vi "VPA QC Print Page.vi"(10 "State Cluster":T1) -> ()   [LabVIEW 2013]
uses:
  Controls/VPA QC General Cluster.ctl
  Controls/VPA QC State Data Cluster.ctl
  Controls/VPA QC State Enum.ctl
  Controls/VPA QC Bool Cluster.ctl
panel:
  out "Cyl B Const":dbl
  out "Cyl A Const.":dbl
  out "Wrap":bool caption="Wrap pump in plastic visqueen."
  out "Clean Water Out":bool caption="Take off the manifold and clear all water out of the\ncylinders and manifold"
  out "Maintenance Hours":bool caption="Reset Maintenance hours from the initial setup menu."
  out "Initialize Pump":bool caption="Initilaize pump to get the top position."
  out "Box":bool caption="Place VPA in box and all other required parts"
  out "Screws":bool caption="Verify that all screws are tight"
  out "Covers":bool caption="Install remaining covers"
  out "Check Fact Rest":bool caption="Go to factory settings and then verify that new constants are still in program"
  out "Volume Calibrated":bool
  out "XDCR Calibrated":bool caption="Match Pressure Transducers"
  out "Verify Pump Operation":bool
  out "XDCR and LS":bool caption="XDCR Set and Limit Switches Tested"
  out "Voltage":bool caption="Ensure pump is running at the voltage specified by customer."
  out "Wired":bool caption="Ensure that VPA is wired correctly."
  out "Tighten Screws":bool
  out "Drive Assem":bool caption="Ensure Drive Assembly checklist is complete."
  out "General Information Clust":T2
  # "VPA Operation Quality Checklist"
  # "Drive Assembly Checklist"
  # "Volume Calibration"
  # "Final Checklist"
  # "XDCR and Limit Switches"
  # "Pump Operation"
  # "Transducers"
  # "Assembly Checklist"
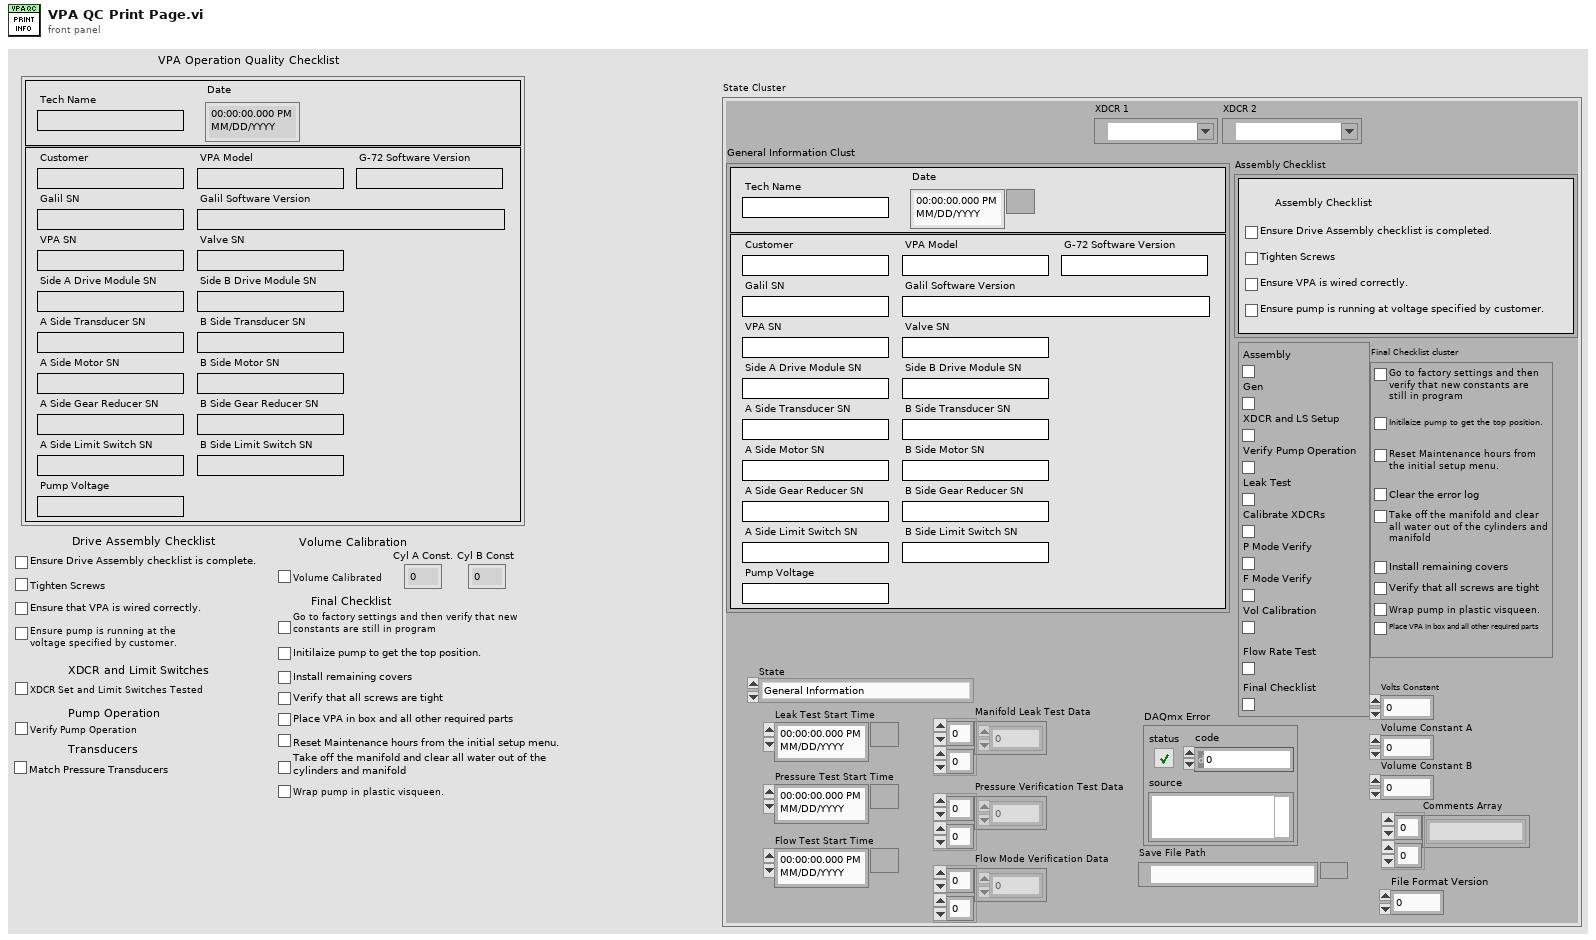
[diagram p1: front panel]
types:
  T1 = typedef "VPA QC State Data Cluster.ctl" = cluster{"XDCR 1":tag, "XDCR 2":tag, "General Information Clust":T2, "Assembly Checklist":cluster{"Ensure Drive Assembly checklist is completed.":bool, "Tighten Screws":bool, "Ensure VPA is wired correctly.":bool, "Ensure pump is running at voltage specified by customer.":bool}, "State":T3, "Manifold Leak Test Data":dbl[][], "Pressure Verification Test Data":dbl[][], "Flow Mode Verification Data":dbl[][], "DAQmx Error":errorcluster, "Bool Cluster":T4, "Leak Test Start Time":timestamp, "Pressure Test Start Time":timestamp, "Flow Test Start Time":timestamp, "Final Checklist cluster":cluster{"Check Fact Rest":bool, "Initialize Pump":bool, "Maintenance Hours":bool, "Clean Water Out":bool, "Covers":bool, "Screws":bool, "Wrap":bool, "Box":bool, "Clear Error Log":bool}, "Volts Constant":dbl, "Volume Constant A":dbl, "Volume Constant B":dbl, "Save File Path":path, "Comments Array":string[][], "File Format Version":u16}
  T2 = typedef "VPA QC General Cluster.ctl" = cluster{"Tech Name":string, "Date":timestamp, "Customer":string, "VPA Model":string, "G-72 Software Version":string, "Galil SN":string, "Galil Software Version":string, "VPA SN":string, "Valve SN":string, "Side A Drive Module SN":string, "Side B Drive Module SN":string, "A Side Transducer SN":string, "B Side Transducer SN":string, "A Side Motor SN":string, "B Side Motor SN":string, "A Side Gear Reducer SN":string, "B Side Gear Reducer SN":string, "A Side Limit Switch SN":string, "B Side Limit Switch SN":string, "Pump Voltage":string}
  T3 = typedef "VPA QC State Enum.ctl" = enum16{"General Information", "XDCR and LS Check", "Check Pump Function", "Manifold/Cylinder Leak Test", "Exit"}
  T4 = typedef "VPA QC Bool Cluster.ctl" = cluster{"Assembly":bool, "Gen":bool, "XDCR and LS Setup":bool, "Verify Pump Operation":bool, "Leak Test":bool, "Calibrate XDCRs":bool, "P Mode Verify":bool, "F Mode Verify":bool, "Vol Calibration":bool, "Flow Rate Test":bool, "Final Checklist":bool}
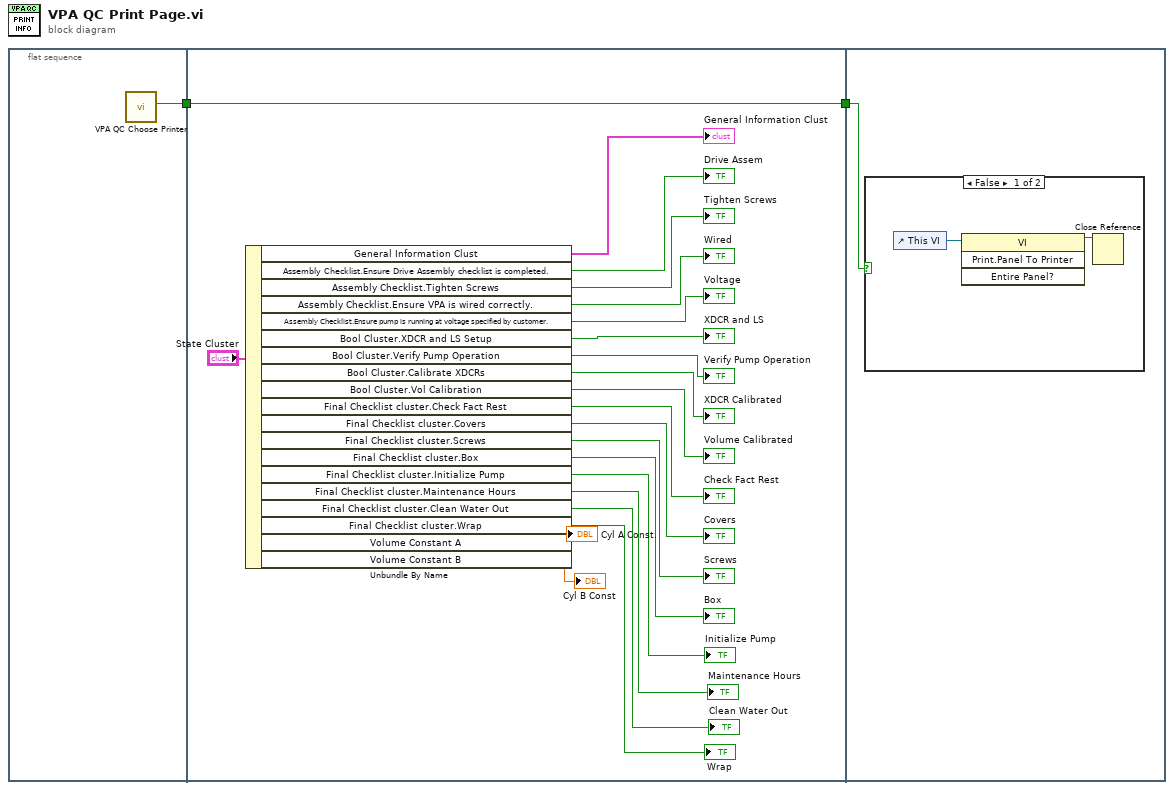
[diagram p0: block diagram]
diagram:
  n1 = flat-sequence {
    tunnel: [w3] -> w1
    tunnel: [w10] -> w2
    tunnel: w1 -> [w10]
    tunnel: w2 -> [w25]
    frame #0 {
      n2 = call "VPA QC Choose Printer.vi"() -> ("Cancelled"=w3:bool)  [unwired: 11 in]
    }
    frame #1 {
      n3 = Unbundle By Name("State Cluster") -> ("General Information Clust"=→"General Information Clust":T2, "Assembly Checklist.Ensure Drive Assembly checklist is completed."=→"Drive Assem":bool, "Assembly Checklist.Tighten Screws"=→"Tighten Screws":bool, "Assembly Checklist.Ensure VPA is wired correctly."=→"Wired":bool, "Assembly Checklist.Ensure pump is running at voltage specified by customer."=→"Voltage":bool, "Bool Cluster.XDCR and LS Setup"=→"XDCR and LS":bool, "Bool Cluster.Verify Pump Operation"=→"Verify Pump Operation":bool, "Bool Cluster.Calibrate XDCRs"=→"XDCR Calibrated":bool, "Bool Cluster.Vol Calibration"=→"Volume Calibrated":bool, "Final Checklist cluster.Check Fact Rest"=→"Check Fact Rest":bool, "Final Checklist cluster.Covers"=→"Covers":bool, "Final Checklist cluster.Screws"=→"Screws":bool, "Final Checklist cluster.Box"=→"Box":bool, "Final Checklist cluster.Initialize Pump"=→"Initialize Pump":bool, "Final Checklist cluster.Maintenance Hours"=→"Maintenance Hours":bool, "Final Checklist cluster.Clean Water Out"=→"Clean Water Out":bool, "Final Checklist cluster.Wrap"=→"Wrap":bool, "Volume Constant A"=→"Cyl A Const.":dbl, "Volume Constant B"=→"Cyl B Const":dbl)
    }
    frame #2 {
      n4 = case shown="False" w25 {
        frame False {
          n5 = control-ref of="This VI"() -> (w27:refnum<vi>)
          n6 = invoke class="VI" method="Print.Panel To Printer"(reference=w27) -> (reference out=w26:refnum<vi>)  [unwired: 3 in, 3 out]
          n7 = Close Reference(reference=w26) -> ()  [unwired: 1 in, 1 out]
        }
        frame True {
        }
      }
    }
  }
